vi "OAT Compensate Vector Data (1 Channel).vi"(0 "magnitudes [RMS]":T2(array[cluster]) {"magnitude" format="%.2f"; "time/rev/rpm" format="%.2f"}, 2 "reset? (F)":bool, 5 "phases [phase lag]":cluster{"time/rev/rpm":dbl[], "phase":dbl[]}[](array[cluster]) {"phase" format="%.2f"; "time/rev/rpm" format="%.2f"}, 7 "vector references":cdb[](array[numeric]) format="%.2f", 11 "error in (no error)":errorcluster, 13 "view info":T1={"dB on? (F)"=FALSE, "unwrap phase? (T)"=TRUE, "unit in degree? (T)"=TRUE}) -> (4 "compensated magnitudes [RMS]":T2(array[cluster]) {"magnitude" format="%.2f"; "time/rev/rpm" format="%.2f"}, 6 "compensated phases [phase lag]":cluster{"time/rev/rpm":dbl[], "phase":dbl[]}[](array[cluster]) {"phase" format="%.2f"; "time/rev/rpm" format="%.2f"}, 8 "actual vector references":cdb[](array[numeric]) format="%.2f", 15 "error out":errorcluster)   [LabVIEW 2017, in "SoundVib_RefDataProcess.lvlib"]
doc: "Compensates for the shaft bow and electrical variations in displacement transducer signals. This VI performs slow-roll compensation by subtracting <B>vector references</B> from the corresponding <B>magnitudes [RMS]</B> and <B>phases [phase lag]</B>. Wire data to the <B>magnitudes [RMS]</B> and <B>phases [phase lag]</B> inputs to determine the polymorphic instance to use or manually select the instance."
uses:
  <vilib>/addons/Sound and Vibration/Order Analysis/Referece Data Processing/SoundVib_RefDataProcess.lvlib
  <vilib>/addons/Sound and Vibration/Order Analysis/Misc/OAT Convert Phase (1 channel).vi
  <vilib>/Analysis/NI_AALPro.lvlib
  <vilib>/addons/Sound and Vibration/Order Analysis/Resample Order Tracking/SoundVib_Resampling.lvlib
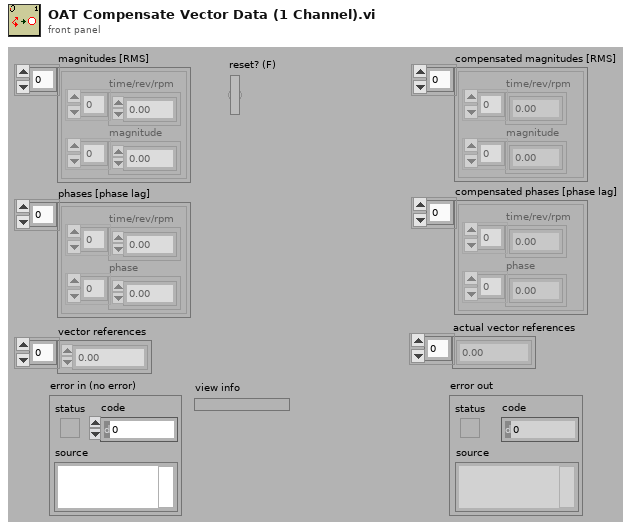
[diagram p1: front panel]
types:
  T1 = cluster{"dB on? (F)":bool, "unwrap phase? (T)":bool, "unit in degree? (T)":bool}
  T2 = cluster{"time/rev/rpm":dbl[], "magnitude":dbl[]}[]
  T3 = cluster{"unwrap phase? (T)":bool, "unit in degree? (T)":bool}
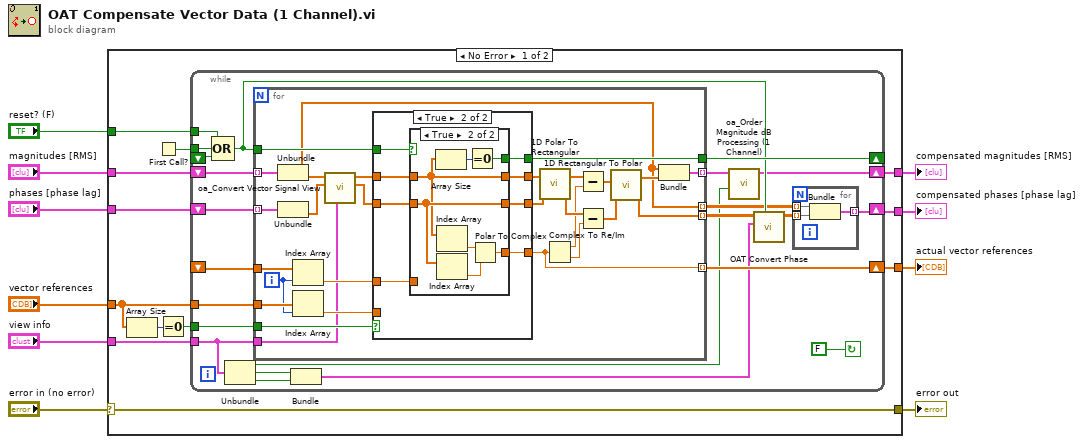
[diagram p0: block diagram]
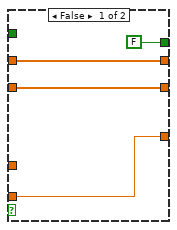
[diagram p2: hidden frame]
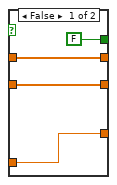
[diagram p3: hidden frame]
diagram:
  n1 = case shown="No Error" "error in (no error)" {
    selector: "error in (no error)" -> [w12 w103]
    tunnel: "magnitudes [RMS]" -> [w17 w102]
    tunnel: "phases [phase lag]" -> [w22 w101]
    tunnel: "vector references" -> [w14 w100]
    tunnel: [w21 w102] -> w7
    tunnel: [w20 w101] -> w6
    tunnel: [w12 w103] -> w4
    tunnel: [w19 w100] -> w3
    tunnel: "view info" -> [w16 _]
    tunnel: "reset? (F)" -> [w11 _]
    frame No Error {
      n2 = Array Size(array=w14) -> (size(s)=w18:i32)
      n3 = First Call?() -> (First Call?: T/F=w13:bool)
      n4 = Equal To 0?(x=w18) -> (x = 0?=w15:bool)
      n5 = while {
        shift-right: [w42] -> w19
        shift-left: _ -> [w41]
        tunnel: w16 -> [w29]
        tunnel: w15 -> [w40]
        tunnel: w14 -> [w39]
        shift-right: [w38] -> _
        shift-left: _ -> [w37]
        tunnel: w13 -> [w36]
        tunnel: w11 -> [w35]
        shift-right: [w24] -> w21
        shift-left: w17 -> [w44]
        shift-right: [w30] -> w20
        shift-left: w22 -> [w43]
        stop <- FALSE continue-if-true
        n6 = Compound Arithmetic op=OR(w35, w36, w37) -> (w33:bool)
        n7 = Unbundle(w29) -> ("dB on? (F)"=w23:bool, "unwrap phase? (T)"=w28:bool, "unit in degree? (T)"=w27:bool)
        n8 = for {
          tunnel: w44 -> [w76] mode=indexing
          tunnel: w43 -> [w75] mode=indexing
          tunnel: [w74] -> w25 mode=indexing
          tunnel: [w64] -> w42 mode=indexing
          tunnel: w41 -> [w63]
          tunnel: w33 -> [w56]
          tunnel: w29 -> [w52]
          tunnel: w40 -> [w59]
          tunnel: w39 -> [w61]
          tunnel: [w57] -> w38
          tunnel: [w55] -> w34 mode=indexing
          tunnel: [w54] -> w31 mode=indexing
          i -> [w60]
          n9 = Unbundle(w76) -> ("time/rev/rpm"=w54:dbl[], "magnitude"=w51:dbl[])
          n10 = Unbundle(w75) -> ("phase out"=w53:dbl[])  [unwired: 1 out]
          n11 = Index Array(array=w63, index=w60) -> (element=w62:cdb)
          n12 = Index Array(array=w61, index=w60) -> (element=w58:cdb)
          n13 = call <vilib>:"oa_Convert Vector Signal View.vi"("view"=w52, "phase"=w53, "magnitude"=w51) -> ("phase out"=w49:dbl[], "magnitude out"=w50:dbl[])  [unwired: 7 in]
          n14 = case shown="True" w59 {
            tunnel: w56 -> [_ w88]
            tunnel: w50 -> [w78 w87]
            tunnel: [w78 w86] -> w73
            tunnel: [w79 w85] -> w72
            tunnel: w49 -> [w79 w84]
            tunnel: [w80 w83] -> w64
            tunnel: w62 -> [_ w82]
            tunnel: w58 -> [w80 _]
            tunnel: [FALSE w81] -> w57
            frame False {
            }
            frame True {
              n15 = case shown="True" w88 {
                tunnel: w87 -> [w91 w95]
                tunnel: [w92 w96] -> w83
                tunnel: w84 -> [w90 w99]
                tunnel: w82 -> [w92 _]
                tunnel: [w91 w95] -> w86
                tunnel: [w90 w99] -> w85
                tunnel: [FALSE w93] -> w81
                frame False {
                }
                frame True {
                  n16 = Array Size(array=w95) -> (size(s)=w94:i32)
                  n17 = Index Array(array=w95) -> (element=w98:dbl)  [unwired: 1 in]
                  n18 = Index Array(array=w99) -> (element=w97:dbl)  [unwired: 1 in]
                  n19 = Equal To 0?(x=w94) -> (x = 0?=w93:bool)
                  n20 = Polar To Complex(1:w97, 2:w98) -> (0:w96:cdb)
                }
              }
            }
          }
          n21 = call <vilib>:"1D Polar To Rectangular.vi"("Magnitude"=w73, "Phase"=w72) -> ("X"=w71:dbl[], "Y"=w70:dbl[])  [unwired: 1 out]
          n22 = Complex To Re/Im(x + iy=w64) -> (x=w66:dbl, y=w65:dbl)
          n23 = Subtract(x=w71, y=w66) -> (x-y=w69:dbl[])
          n24 = Subtract(x=w70, y=w65) -> (x-y=w68:dbl[])
          n25 = call <vilib>:"1D Rectangular To Polar.vi"("X"=w69, "Y"=w68) -> ("Magnitude"=w67:dbl[], "Phase"=w55:dbl[])  [unwired: 1 out]
          n26 = Bundle("time/rev/rpm"=w54, "Magnitude"=w67) -> (w74:cluster{"time/rev/rpm":dbl[], "Magnitude":dbl[]})  [unwired: 1 in]
        }
        n27 = Bundle("unwrap phase? (T)"=w28, "unit in degree? (T)"=w27) -> (w26:T3)  [unwired: 1 in]
        n28 = call <vilib>:"oa_Order Magnitude dB Processing (1 Channel).vi"("dB on? (T)"=w23, "magnitudes"=w25) -> ("magnitudes dB"=w24:T2)  [unwired: 9 in]
        n29 = call-poly <vilib>:"OAT Convert Phase.vi"("reset (TRUE)"=w33, "desired phase setting"=w26, "phase in (rad)"=w34) -> ("phase out"=w32:dbl[][])  [unwired: 8 in]
        n30 = for {
          tunnel: w32 -> [w47] mode=indexing
          tunnel: w31 -> [w48] mode=indexing
          tunnel: [w46] -> w30 mode=indexing
          n31 = Bundle("time/rev/rpm"=w48, "phase out"=w47) -> (w46:cluster{"time/rev/rpm":dbl[], "phase out":dbl[]})  [unwired: 1 in]
        }
      }
    }
    frame Error {
    }
  }
  "error out" <- w4
  "compensated magnitudes [RMS]" <- w7
  "compensated phases [phase lag]" <- w6
  "actual vector references" <- w3
